vi "Read and Update Metadata.vi"(8 "error in (no error)":errorcluster, 11 "Update Metadata":bool) -> (0 "error out":errorcluster, 3 "Plugin Info":T1[](array[typedef]))   [LabVIEW 2021, in "CIFPluginLoader.lvclass"]
uses:
  CIFPluginLoader.lvclass
  Common/typedef/Discovered Plugin.ctl
  <vilib>/CIF Foundation/CIF Core/CIFCore/Common/Typedef/Version.ctl
  Common/typedef/Plugin Metadata.ctl
  Common/typedef/Loader Type.ctl
  <vilib>/CIF Foundation/CIF Core/CIFUtilities/CIFConfigurationFile/typedef/Location Type.ctl
  CIFPluginLoader.lvclass/CIFPluginLoader.ctl
  <vilib>/CIF Foundation/CIF Core/CIFUtilities/CIFConfigurationFile/CIF Configuration File.lvlib
  <vilib>/Utility/config.llb/NI_LVConfig.lvlib
  <vilib>/CIF Foundation/CIF Core/CIFCore/Common/CIFCoreCommon.lvlib
  Common/Manager Common.lvlib
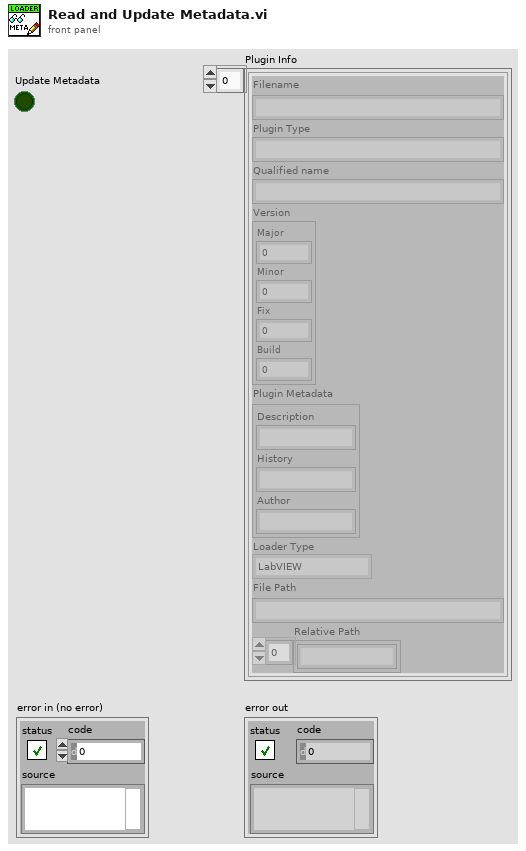
[diagram p1: front panel]
types:
  T1 = typedef "Manager Common.lvlib/Discovered Plugin.ctl" = cluster{"Filename":string, "Plugin Type":string, "Qualified name":string, "Version":T2, "Plugin Metadata":T3, "Loader Type":T4, "File Path":string, "Relative Path":string[]}
  T2 = typedef "CIFCoreCommon.lvlib/Version.ctl" = cluster{"Major":i32, "Minor":i32, "Fix":i32, "Build":i32}
  T3 = typedef "Manager Common.lvlib/Plugin Metadata.ctl" = cluster{"Description":string, "History":string, "Author":string}
  T4 = typedef "Manager Common.lvlib/Loader Type.ctl" = enum16{"LabVIEW"}
  T5 = typedef "CIF Configuration File.lvlib/Location Type.ctl" = enum8{"Config File", "Manager", "Protos", "Plugins", "UI Plugins", "Logs", "Orchestrations", "Loaders"}
  T6 = typedef "NI_LVConfig.lvlib/Config Data RefNum.ctl" = refnum<k1>
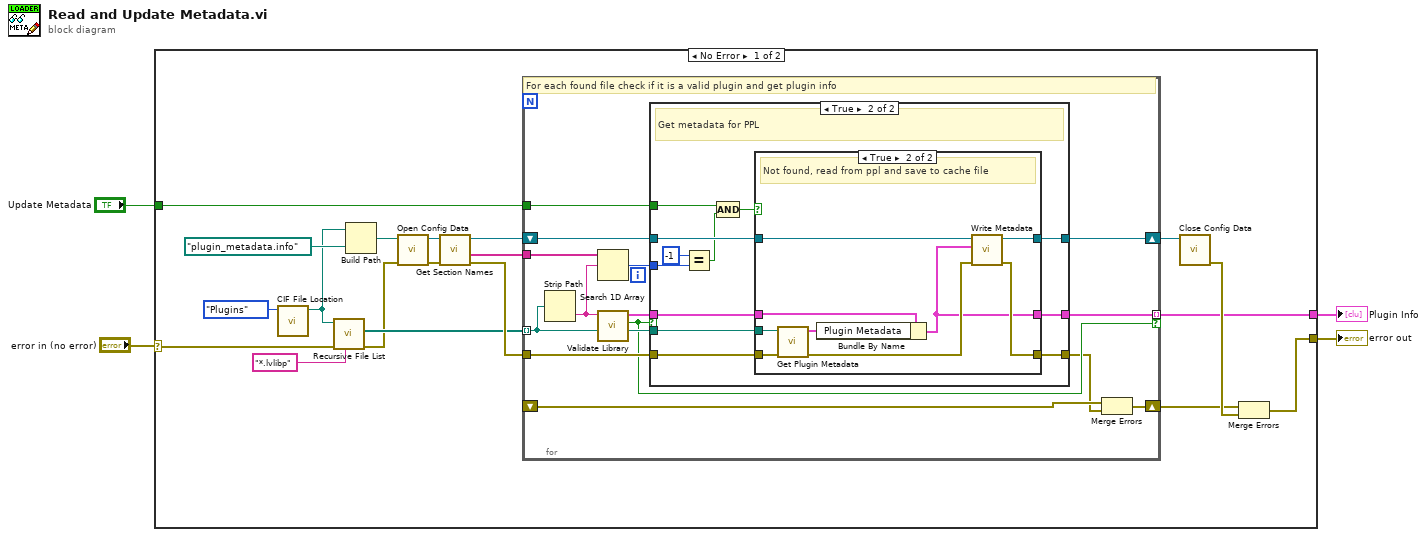
[diagram p0: block diagram]
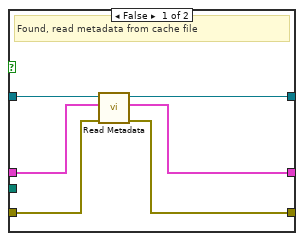
[diagram p3: hidden frame]
diagram:
  n1 = case shown="No Error" "error in (no error)" {
    selector: "error in (no error)" -> [w8 w69]
    tunnel: [w13 w69] -> w4
    tunnel: "Update Metadata" -> [w12 _]
    tunnel: [w6 _] -> w1
    frame No Error {
      n2 = call <vilib>:"CIF File Location.vi"("LocationType"=Location_Type."Plugins") -> ("Location"=w11:path)  [unwired: 10 in]
      n3 = call <vilib>:"Recursive File List.vi"("pattern"="*.lvlibp", "error in (no error)"=w8, "Folder Path"=w11) -> ("error out"=w7:errorcluster, "All Files in Dir"=w9:path[])  [unwired: 4 in, 3 out]
      n4 = Build Path(base path=w11, name or relative path=path "plugin_metadata.info") -> (appended path=w22:path)
      n5 = call <vilib>:"Open Config Data.vi"("error in (no error)"=w7, "configuration file path"=w22) -> ("error out"=w18:errorcluster, "refnum"=w19:T6)  [unwired: 7 in, 1 out]
      n6 = call <vilib>:"Get Section Names.vi"("error in (no error)"=w18, "refnum"=w19) -> ("error out"=w16:errorcluster, "section names"=w15:string[], "refnum out"=w17:T6)  [unwired: 7 in]
      n7 = for {
        tunnel: [w29] -> w6 mode=indexing if=w31
        tunnel: w16 -> [w38]
        shift-right: [w36] -> w20
        shift-left: w17 -> [w37]
        tunnel: w15 -> [w35]
        tunnel: w12 -> [w30]
        tunnel: w9 -> [w28] mode=indexing
        shift-right: [w26] -> w5
        shift-left: _ -> [w25]
        # "For each found file check if it is a valid plugin and get plugin info"
        n8 = Strip Path(path=w28) -> (name=w27:string)  [unwired: 1 out]
        n9 = Search 1D Array(1D array=w35, element=w27) -> (index of element=w33:i32)  [unwired: 1 in]
        n10 = call "Validate Library.vi"("path in"=w28, "Filename"=w27) -> ("path (dup)"=w32:path, "valid"=w31:bool, "Discovered Plugin"=w34:T1)  [unwired: 7 in]
        n11 = case shown="True" w31 {
          tunnel: w34 -> [w40 w43]
          tunnel: w32 -> [_ w53]
          tunnel: w38 -> [w41 w52]
          tunnel: [w40 w42] -> w29
          tunnel: [w41 w49] -> w24
          tunnel: w37 -> [w39 w51]
          tunnel: [w39 w50] -> w36
          tunnel: w33 -> [_ w48]
          tunnel: w30 -> [_ w46]
          frame False {
            # "Invalid"
          }
          frame True {
            # "Get metadata for PPL"
            n12 = Equal?(x=-1, y=w48) -> (x = y?=w45:bool)
            n13 = Compound Arithmetic op=AND(w46, w45) -> (w44:bool)
            n14 = case shown="True" w44 {
              tunnel: w43 -> [w58 w60]
              tunnel: w53 -> [_ w68]
              tunnel: w52 -> [w55 w66]
              tunnel: w51 -> [w59 w65]
              tunnel: [w56 w64] -> w50
              tunnel: [w57 w61] -> w42
              tunnel: [w54 w62] -> w49
              frame False {
                # "Found, read metadata from cache file"
                n15 = call "Read Metadata.vi"("error in (no error)"=w55, "Plugin Info in"=w58, "metadata ref in"=w59) -> ("error out"=w54:errorcluster, "Plugin Info out"=w57:T1, "metadata ref dup"=w56:T6)  [unwired: 6 in]
              }
              frame True {
                # "Not found, read from ppl and save to cache file"
                n16 = call "Get Plugin Metadata.vi"("error in (no error)"=w66, "Packed Library Path"=w68) -> ("error out"=w63:errorcluster, "Plugin Metadata"=w67:T3)  [unwired: 8 in]
                n17 = Bundle By Name(cluster=w60, "Plugin Metadata"=w67) -> (w61:T1)
                n18 = call "Write Metadata.vi"("error in (no error)"=w63, "Plugin Info"=w61, "metadata ref in"=w65) -> ("error out"=w62:errorcluster, "metadata ref dup"=w64:T6)  [unwired: 7 in]
              }
            }
          }
        }
        n19 = Merge Errors(w25, w24) -> (w26:errorcluster)
      }
      n20 = call <vilib>:"Close Config Data.vi"("refnum"=w20) -> ("error out"=w14:errorcluster)  [unwired: 9 in, 1 out]
      n21 = Merge Errors(w5, w14) -> (w13:errorcluster)
    }
    frame Error {
    }
  }
  "error out" <- w4
  "Plugin Info" <- w1
